vi "TL behavior S-Wall.vi"(1 "Behavior\nVelocity":dbl, 2 "Activate?":bool=TRUE, 3 "Sensor":T1) -> (0 "S-Wall Array":dbl[](array[numeric]))   [LabVIEW 2014]
uses:
  sensorsSTD.ctl
panel:
  out "Waveform Graph":cluster{dbl, dbl, dbl[]}(graph)
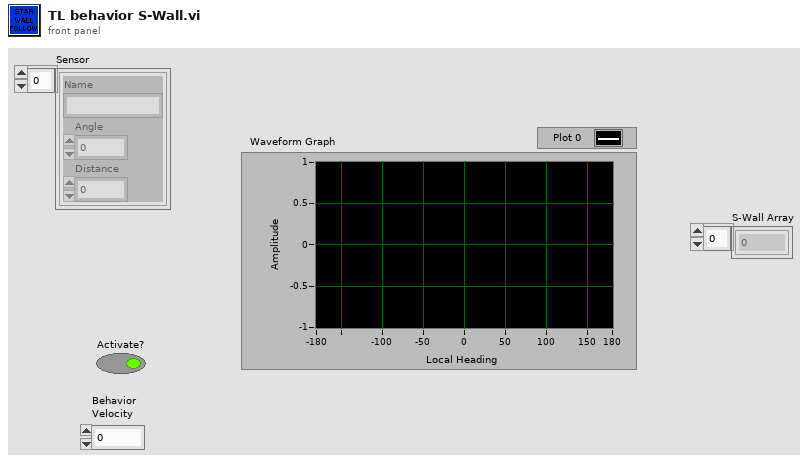
[diagram p1: front panel]
types:
  T1 = typedef "sensorsSTD.ctl" = cluster{"Name":string, "Angle":dbl, "Distance":dbl}[]
  T2 = cluster{"Name":string, "Angle":dbl, "Distance":dbl}
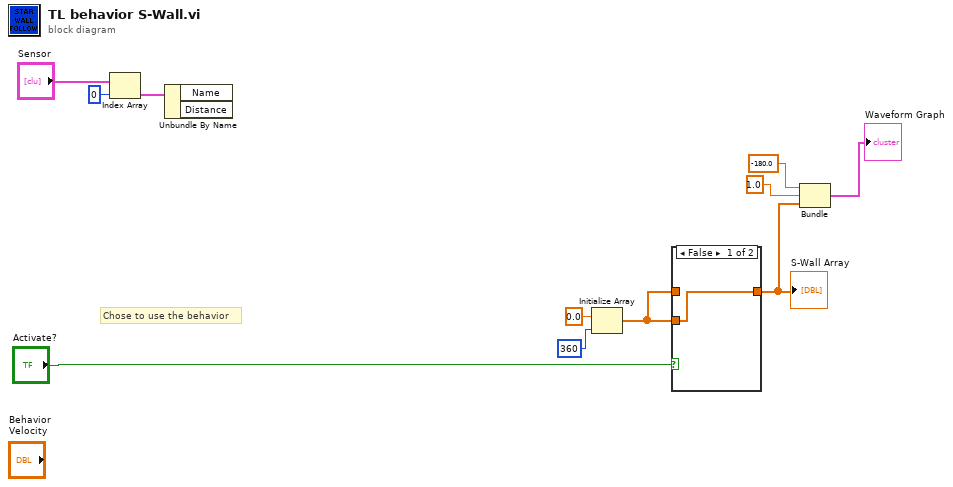
[diagram p0: block diagram]
diagram:
  # "Chose to use the behavior"
  n1 = Index Array(array="Sensor", index=0) -> (element=w9:T2)
  n2 = Unbundle By Name(w9) -> ()  [unwired: 2 out]
  n3 = Initialize Array(0.0 ("element"), 360 ("dimension size")) -> (w2:dbl[])
  n4 = case shown="False" "Activate?" {
    tunnel: w2 -> [w12 _]
    tunnel: w2 -> [_ w13]
    tunnel: [w12 w13] -> w1
    frame False {
    }
    frame True {
    }
  }
  "S-Wall Array" <- w1
  n5 = Bundle(-180.0, 1.0, w1) -> (→"Waveform Graph":cluster{dbl, dbl, dbl[]})  [unwired: 1 in]
